vi "Destroy.vi"(8 "error in (no error)":errorcluster, 11 "CameraTool Class in":refnum<class "CameraTool Class.lvclass">) -> (0 "error out":errorcluster, 3 "CameraTool Class out":refnum<class "CameraTool Class.lvclass">)   [LabVIEW 2011, in "CameraTool Class.lvclass"]
uses:
  CameraTool Class.lvclass
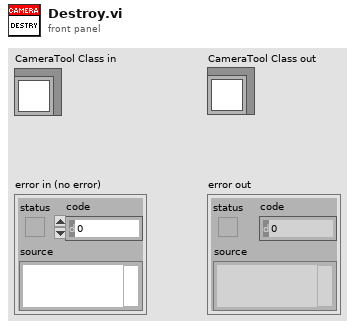
[diagram p1: front panel]
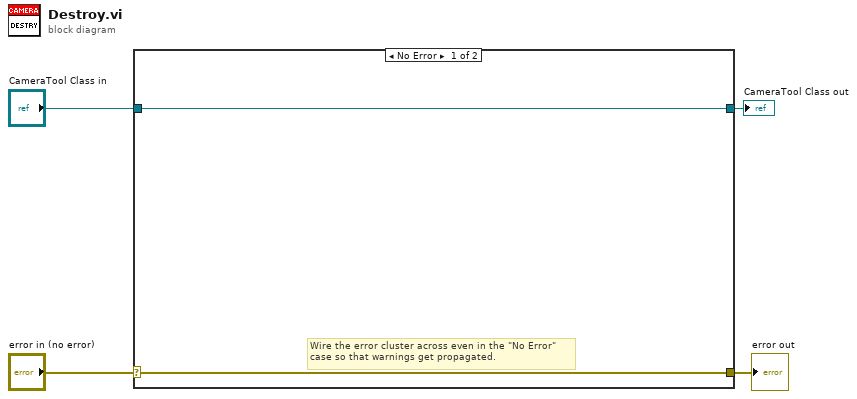
[diagram p0: block diagram]
diagram:
  n1 = case shown="No Error" "error in (no error)" {
    selector: "error in (no error)" -> [w5 w8]
    tunnel: [w5 w8] -> w3
    tunnel: [w6 w7] -> w1
    tunnel: "CameraTool Class in" -> [w6 w7]
    frame No Error {
      # "Wire the error cluster across even in the \"No Error\"\ncase so that warnings get propagated."
    }
    frame Error {
    }
  }
  "error out" <- w3
  "CameraTool Class out" <- w1
